vi "postSubDataUE.vi"(6 "newValue (T)":bool=TRUE, 8 "error in (no error)":errorcluster, 9 "value":variant, 10 "subDataSV":T1, 11 "PubSubDataEvent in":refnum<class "PubSubDataEvent.lvclass">) -> (0 "error out":errorcluster, 3 "PubSubDataEvent out":refnum<class "PubSubDataEvent.lvclass">)   [LabVIEW 2016, in "PubSubDataEvent.lvclass"]
uses:
  PubSubDataEvent.lvclass
  Typedefs/SubDataSignal.ctl
  PubSubDataEvent.lvclass/PubSubDataEvent.ctl
  ts_sallv_sedspectrometer/DataTypes/command_disable.ctl
  ts_sallv_sedspectrometer/DataTypes/command_enable.ctl
  ts_sallv_sedspectrometer/DataTypes/command_exitControl.ctl
  ts_sallv_sedspectrometer/DataTypes/command_standby.ctl
  ts_sallv_sedspectrometer/DataTypes/logevent_Heartbeat.ctl
  ts_sallv_sedspectrometer/DataTypes/command_start.ctl
  ts_sallv_sedspectrometer/DataTypes/command_captureSpectImage.ctl
  ts_sallv_sedspectrometer/DataTypes/command_setSpectTempSetpoint.ctl
  ts_sallv_sedspectrometer/DataTypes/command_stopImageCapture.ctl
  ts_sallv_sedspectrometer/SALLV_sedSpectrometer.lvlib
  Typedefs/SEDSpectrometerTypedefs.lvlib
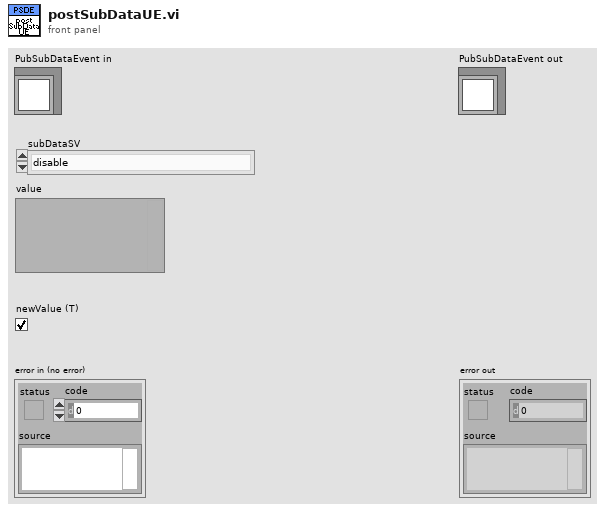
[diagram p1: front panel]
types:
  T1 = typedef "SEDSpectrometerTypedefs.lvlib/SubDataSignal.ctl" = enum16{"disable", "enable", "exit", "standby", "HeartbeatIn", "start", "captureSpectImage", "setSpectTempSetpoint", "stopImageCapture"}
  T2 = typedef "TypedefsDataEvents.lvlib/SubDataEvents.ctl" = cluster{"disable":refnum<user-event>, "enable":refnum<user-event>, "exitControl":refnum<user-event>, "standby":refnum<user-event>, "heartbeat":refnum<user-event>, "start":refnum<user-event>, "captureSpectImage":refnum<user-event>, "setSpectTempSetpoint":refnum<user-event>, "stopImageCapture":refnum<user-event>}
  T3 = typedef "SALLV_sedSpectrometer.lvlib/command_disable.ctl" = cluster{"disable":bool}
  T4 = typedef "SALLV_sedSpectrometer.lvlib/command_enable.ctl" = cluster{"enable":bool}
  T5 = typedef "SALLV_sedSpectrometer.lvlib/command_exitControl.ctl" = cluster{"exitControl":bool}
  T6 = typedef "SALLV_sedSpectrometer.lvlib/command_standby.ctl" = cluster{"standBy":bool}
  T7 = typedef "SALLV_sedSpectrometer.lvlib/logevent_Heartbeat.ctl" = cluster{"heartbeat":bool, "priority":i32}
  T8 = typedef "SALLV_sedSpectrometer.lvlib/command_start.ctl" = cluster{"settingsToApply":string}
  T9 = typedef "SALLV_sedSpectrometer.lvlib/command_captureSpectImage.ctl" = cluster{"spectId":u16, "intTime":sgl, "intDelay":dbl, "numAverages":u16, "numScans":i32, "type":string, "lamp":string}
  T10 = typedef "SALLV_sedSpectrometer.lvlib/command_setSpectTempSetpoint.ctl" = cluster{"spectId":u16, "setpoint":sgl}
  T11 = typedef "SALLV_sedSpectrometer.lvlib/command_stopImageCapture.ctl" = cluster{"SpectId":u16}
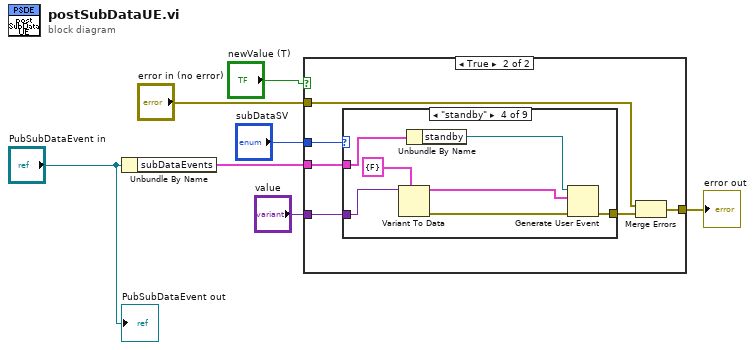
[diagram p0: block diagram]
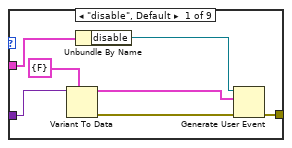
[diagram p3: hidden frame]
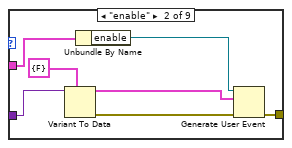
[diagram p4: hidden frame]
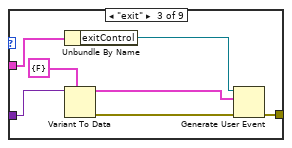
[diagram p5: hidden frame]
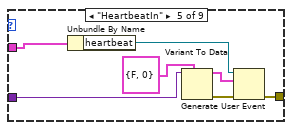
[diagram p6: hidden frame]
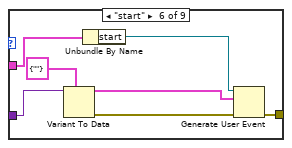
[diagram p7: hidden frame]
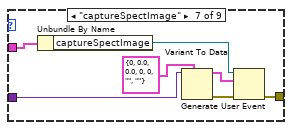
[diagram p8: hidden frame]
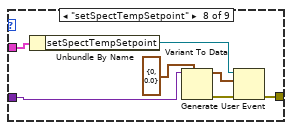
[diagram p9: hidden frame]
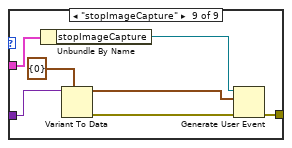
[diagram p10: hidden frame]
diagram:
  n1 = Unbundle By Name("PubSubDataEvent in") -> ("subDataEvents"=w5:T2)
  n2 = case shown="True" "newValue (T)" {
    tunnel: w5 -> [_ w13]
    tunnel: "subDataSV" -> [_ w14]
    tunnel: "value" -> [_ w12]
    tunnel: "error in (no error)" -> [w8 w10]
    tunnel: [w8 w9] -> w3
    frame False {
    }
    frame True {
      n3 = case shown="\"standby\"" w14 {
        tunnel: w13 -> [w21 w28 w35 w42 w49 w56 w63 w65 w75]
        tunnel: w12 -> [w20 w27 w34 w41 w48 w55 w61 w67 w72]
        tunnel: [w17 w24 w30 w38 w45 w52 w57 w66 w71] -> w11
        frame "disable", Default {
          n4 = Variant To Data(type=T3 {"disable"=FALSE} ("event data"), Variant=w20) -> (data=w16:T3, error out=w18:errorcluster)  [unwired: 1 in]
          n5 = Unbundle By Name(w21) -> ("disable"=w19:refnum<user-event>)
          n6 = Generate User Event(user event=w19, event data cluster=w16, error in=w18) -> (error out=w17:errorcluster)  [unwired: 1 in, 1 out]
        }
        frame "enable" {
          n7 = Variant To Data(type=T4 {"enable"=FALSE} ("event data"), Variant=w27) -> (data=w23:T4, error out=w25:errorcluster)  [unwired: 1 in]
          n8 = Unbundle By Name(w28) -> ("enable"=w26:refnum<user-event>)
          n9 = Generate User Event(user event=w26, event data cluster=w23, error in=w25) -> (error out=w24:errorcluster)  [unwired: 1 in, 1 out]
        }
        frame "exit" {
          n10 = Unbundle By Name(w35) -> ("exitControl"=w33:refnum<user-event>)
          n11 = Variant To Data(type=T5 {"exitControl"=FALSE} ("event data"), Variant=w34) -> (data=w32:T5, error out=w31:errorcluster)  [unwired: 1 in]
          n12 = Generate User Event(user event=w33, event data cluster=w32, error in=w31) -> (error out=w30:errorcluster)  [unwired: 1 in, 1 out]
        }
        frame "standby" {
          n13 = Variant To Data(type=T6 {"standBy"=FALSE} ("event data"), Variant=w41) -> (data=w36:T6, error out=w39:errorcluster)  [unwired: 1 in]
          n14 = Unbundle By Name(w42) -> ("standby"=w40:refnum<user-event>)
          n15 = Generate User Event(user event=w40, event data cluster=w36, error in=w39) -> (error out=w38:errorcluster)  [unwired: 1 in, 1 out]
        }
        frame "HeartbeatIn" {
          n16 = Unbundle By Name(w49) -> ("heartbeat"=w47:refnum<user-event>)
          n17 = Variant To Data(type=T7 {"heartbeat"=FALSE, "priority"=0} ("event data"), Variant=w48) -> (data=w44:T7, error out=w46:errorcluster)  [unwired: 1 in]
          n18 = Generate User Event(user event=w47, event data cluster=w44, error in=w46) -> (error out=w45:errorcluster)  [unwired: 1 in, 1 out]
        }
        frame "start" {
          n19 = Variant To Data(type=T8 {"settingsToApply"=""} ("event data"), Variant=w55) -> (data=w51:T8, error out=w53:errorcluster)  [unwired: 1 in]
          n20 = Unbundle By Name(w56) -> ("start"=w54:refnum<user-event>)
          n21 = Generate User Event(user event=w54, event data cluster=w51, error in=w53) -> (error out=w52:errorcluster)  [unwired: 1 in, 1 out]
        }
        frame "captureSpectImage" {
          n22 = Unbundle By Name(w63) -> ("captureSpectImage"=w60:refnum<user-event>)
          n23 = Variant To Data(type=T9 {"spectId"=0, "intTime"=0.0, "intDelay"=0.0, "numAverages"=0, "numScans"=0, "type"="", "lamp"=""} ("command_CaptureSpectImage"), Variant=w61) -> (data=w59:T9, error out=w58:errorcluster)  [unwired: 1 in]
          n24 = Generate User Event(user event=w60, event data cluster=w59, error in=w58) -> (error out=w57:errorcluster)  [unwired: 1 in, 1 out]
        }
        frame "setSpectTempSetpoint" {
          n25 = Unbundle By Name(w65) -> ("setSpectTempSetpoint"=w64:refnum<user-event>)
          n26 = Variant To Data(type=T10 {"spectId"=0, "setpoint"=0.0} ("command_SetSpectTempSetpoint"), Variant=w67) -> (data=w70:T10, error out=w69:errorcluster)  [unwired: 1 in]
          n27 = Generate User Event(user event=w64, event data cluster=w70, error in=w69) -> (error out=w66:errorcluster)  [unwired: 1 in, 1 out]
        }
        frame "stopImageCapture" {
          n28 = Unbundle By Name(w75) -> ("stopImageCapture"=w74:refnum<user-event>)
          n29 = Variant To Data(type=T11 {"SpectId"=0} ("command_StopImageCapture"), Variant=w72) -> (data=w77:T11, error out=w76:errorcluster)  [unwired: 1 in]
          n30 = Generate User Event(user event=w74, event data cluster=w77, error in=w76) -> (error out=w71:errorcluster)  [unwired: 1 in, 1 out]
        }
      }
      n31 = Merge Errors(w10, w11) -> (w9:errorcluster)
    }
  }
  "error out" <- w3
  "PubSubDataEvent out" <- "PubSubDataEvent in"
